vi "AMZ_S3_APIHLP_Is Bucket name DNS Compliant.vi"(11 "Bucket in":string) -> (2 "DNS Compliant?":bool, 3 "Bucket out":string)   [LabVIEW 2015, in "LV Interface for Amazon S3.lvlib"]
uses:
  LV Interface for Amazon S3.lvlib
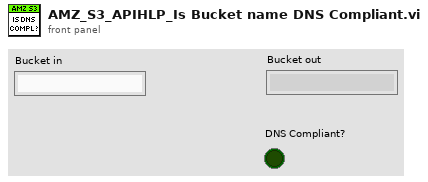
[diagram p1: front panel]
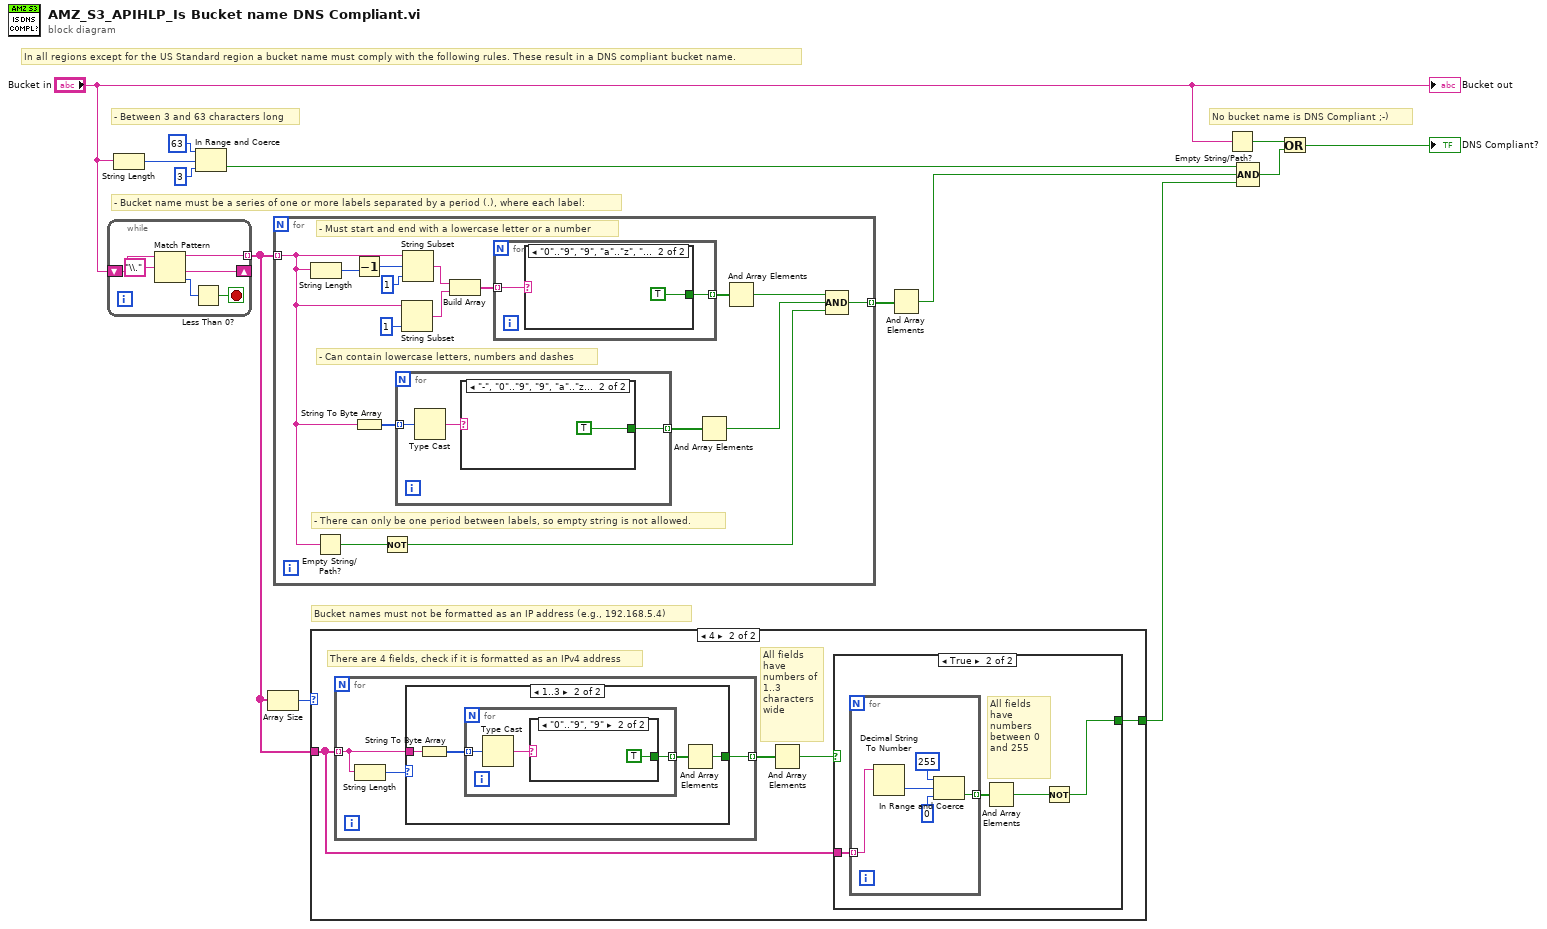
[diagram p0: block diagram]
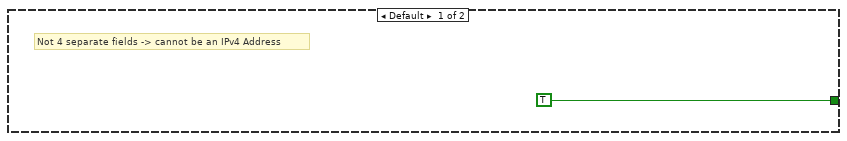
[diagram p2: hidden frame]
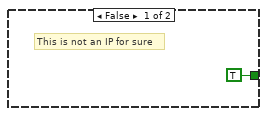
[diagram p3: hidden frame]
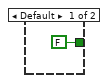
[diagram p4: hidden frame]
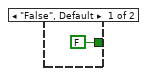
[diagram p5: hidden frame]
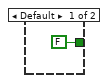
[diagram p6: hidden frame]
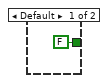
[diagram p7: hidden frame]
diagram:
  # "No bucket name is DNS Compliant ;-)"
  # "Bucket names must not be formatted as an IP address (e.g., 192.168.5.4)"
  # "- Bucket name must be a series of one or more labels separated by a period (.), where each label:"
  # "In all regions except for the US Standard region a bucket name must comply with the following rules. These result in a DNS compliant bucket name."
  # "- Between 3 and 63 characters long"
  n1 = while {
    shift-right: [w17] -> _
    shift-left: "Bucket in" -> [w19]
    tunnel: [w14] -> w1 mode=indexing
    stop <- w15 stop-if-true
    n2 = Match Pattern(string=w19, regular expression="\\.") -> (before substring=w14:string, after substring=w17:string, offset past match=w16:i32)  [unwired: 1 in, 1 out]
    n3 = Less Than 0?(x=w16) -> (x < 0?=w15:bool)
  }
  n4 = String Length(string="Bucket in") -> (length=w11:i32)
  n5 = In Range and Coerce(upper limit=63, x=w11, lower limit=3) -> (In Range?=w8:bool)  [unwired: 1 out]
  n6 = Array Size(array=w1) -> (size(s)=w10:i32)
  n7 = for {
    tunnel: w1 -> [w20] mode=indexing
    tunnel: [w22] -> w9 mode=indexing
    # "- There can only be one period between labels, so empty string is not allowed."
    # "- Can contain lowercase letters, numbers and dashes"
    # "- Must start and end with a lowercase letter or a number"
    n8 = String Length(string=w20) -> (length=w21:i32)
    n9 = Empty String/Path?(string/path=w20) -> (empty?=w26:bool)
    n10 = Decrement(x=w21) -> (x-1=w35:i32)
    n11 = String To Byte Array(string=w20) -> (unsigned byte array=w28:u8[])
    n12 = Not(x=w26) -> (.not. x?=w24:bool)
    n13 = for {
      tunnel: w28 -> [w38] mode=indexing
      tunnel: [w36] -> w27 mode=indexing
      n14 = Type Cast(x=w38) -> (*(type *) &x=w37:string)  [unwired: 1 in]
      n15 = case shown="\"-\", \"0\"..\"9\", \"9\", \"a\"..\"z\", \"z\"" w37 {
        tunnel: [FALSE TRUE] -> w36
        frame Default {
        }
        frame "-", "0".."9", "9", "a".."z", "z" {
        }
      }
    }
    n16 = String Subset(string=w20, length (rest)=1 ("length (rest)")) -> (substring=w31:string)  [unwired: 1 in]
    n17 = String Subset(string=w20, offset (0)=w35, length (rest)=1 ("length (rest)")) -> (substring=w32:string)
    n18 = Build Array(w32, w31) -> (w30:string[])
    n19 = for {
      tunnel: w30 -> [w42] mode=indexing
      tunnel: [w41] -> w29 mode=indexing
      n20 = case shown="\"0\"..\"9\", \"9\", \"a\"..\"z\", \"z\"" w42 {
        tunnel: [FALSE TRUE] -> w41
        frame Default {
        }
        frame "0".."9", "9", "a".."z", "z" {
        }
      }
    }
    n21 = And Array Elements(Boolean array=w27) -> (logical AND=w23:bool)
    n22 = And Array Elements(Boolean array=w29) -> (logical AND=w25:bool)
    n23 = Compound Arithmetic op=AND(w25, w23, w24) -> (w22:bool)
  }
  n24 = case shown="4" w10 {
    tunnel: [TRUE w49] -> w6
    tunnel: w1 -> [_ w46]
    frame Default {
      # "Not 4 separate fields -> cannot be an IPv4 Address"
    }
    frame 4 {
      # "All fields have\nnumbers of 1..3\ncharacters wide"
      # "There are 4 fields, check if it is formatted as an IPv4 address"
      n25 = for {
        tunnel: w46 -> [w61] mode=indexing
        tunnel: [w60] -> w48 mode=indexing
        n26 = String Length(string=w61) -> (length=w62:i32)
        n27 = case shown="1..3" w62 {
          tunnel: w61 -> [_ w67]
          tunnel: [FALSE w64] -> w60
          frame Default {
          }
          frame 1..3 {
            n28 = String To Byte Array(string=w67) -> (unsigned byte array=w66:u8[])
            n29 = for {
              tunnel: w66 -> [w70] mode=indexing
              tunnel: [w68] -> w65 mode=indexing
              n30 = Type Cast(x=w70) -> (*(type *) &x=w69:string)  [unwired: 1 in]
              n31 = case shown="\"0\"..\"9\", \"9\"" w69 {
                tunnel: [FALSE TRUE] -> w68
                frame "False", Default {
                }
                frame "0".."9", "9" {
                }
              }
            }
            n32 = And Array Elements(Boolean array=w65) -> (logical AND=w64:bool)
          }
        }
      }
      n33 = And Array Elements(Boolean array=w48) -> (logical AND=w47:bool)
      n34 = case shown="True" w47 {
        tunnel: [TRUE w51] -> w49
        tunnel: w46 -> [_ w54]
        frame False {
          # "This is not an IP for sure"
        }
        frame True {
          # "All fields have\nnumbers between 0 and 255"
          n35 = for {
            tunnel: w54 -> [w59] mode=indexing
            tunnel: [w55] -> w53 mode=indexing
            n36 = Decimal String To Number(string=w59) -> (number=w58:i32)  [unwired: 2 in, 1 out]
            n37 = In Range and Coerce(upper limit=255, x=w58, lower limit=0) -> (In Range?=w55:bool)  [unwired: 1 out]
          }
          n38 = And Array Elements(Boolean array=w53) -> (logical AND=w52:bool)
          n39 = Not(x=w52) -> (.not. x?=w51:bool)
        }
      }
    }
  }
  n40 = And Array Elements(Boolean array=w9) -> (logical AND=w7:bool)
  n41 = Empty String/Path?(string/path="Bucket in") -> (empty?=w4:bool)
  n42 = Compound Arithmetic op=AND(w8, w7, w6) -> (w3:bool)
  n43 = Or(x=w4, y=w3) -> (x .or. y?=→"DNS Compliant?":bool)
  "Bucket out" <- "Bucket in"
